vi "run on default pool.vi"(10 "results reporter":refnum<class "results reporter.lvclass">, 11 "task":refnum<class "task.lvclass">) -> (0 "error out":errorcluster)   [LabVIEW 2014]
uses:
  results reporter/results reporter.lvclass
  task/task.lvclass
  dispatcher/execution system.ctl
  dispatcher/thread pool.lvclass
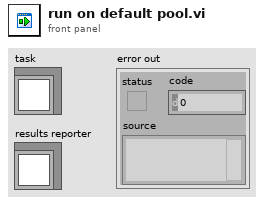
[diagram p1: front panel]
types:
  T1 = typedef "thread pool.lvclass/execution system.ctl" = enum32{"user interface", "standard", "instrument i/o", "data acquisition", "other 1", "other 2"}
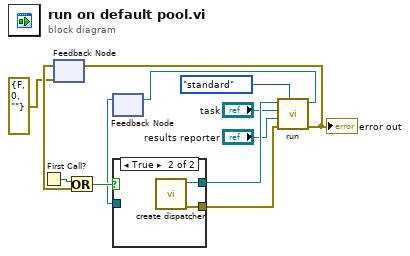
[diagram p0: block diagram]
diagram:
  n1 = First Call?() -> (First Call?: T/F=w10:bool)
  n2 = feedback #1(errorcluster {"status"=FALSE, "code"=0, "source"=""} ("error out")) -> (w8:errorcluster)
  n3 = Or(x=w10, y=w8) -> (x .or. y?=w12:bool)
  n4 = feedback #2() -> (w9:refnum<class "thread pool.lvclass">)  [unwired: 1 in]
  n5 = case shown="True" w12 {
    tunnel: [w13 w15] -> w5
    tunnel: [_ w14] -> w11
    tunnel: w9 -> [w13 _]
    frame False {
    }
    frame True {
      n6 = call "create dispatcher.vi"() -> ("error out"=w14:errorcluster, "dispatcher"=w15:refnum<class "thread pool.lvclass">)  [unwired: 10 in]
    }
  }
  n7 = call "run.vi"("execution system"=execution_system."standard", "error in"=w11, "results reporter"="results reporter", "task"="task", "thread pool in"=w5) -> ("error out"=w6:errorcluster, "thread pool out"=w4:refnum<class "thread pool.lvclass">)  [unwired: 5 in]
  "error out" <- w6
  n8 = feedback-in #1(w6) -> ()
  n9 = feedback-in #2(w4) -> ()
